vi "Agilent B2900oP AND ip.vi"() -> ()   [LabVIEW 2017]
doc: "This example shows how to configure the instrument's output voltage level, over current protection, and over voltage protection. The actual voltage level and actual current level are returned as well as whether over voltage protection (OVP) or over current protection (OCP) has been tripped."
uses:
  <instrlib>/Agilent B2900 Series/Agilent B2900 Series.lvlib
panel:
  in  "Compliance Voltage (2 V)":dbl=2.0 format="%#_13g"
  in  "Source current (A)":dbl
  in  "Source Range (A)":dbl=2.0
  in  "Enable Output Protection (T: Enable)":bool=TRUE
  in  "Stop":bool
  out "Actual Current Level (A)":dbl format="%_6g"
  out "Actual Voltage Level (V)":dbl format="%_6g"
  in  "VISA resource name":refnum<visa-resource-name>
  # "Compliance Protection"
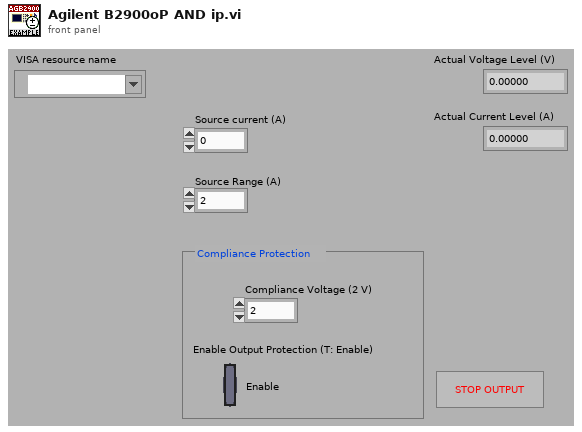
[diagram p1: front panel]
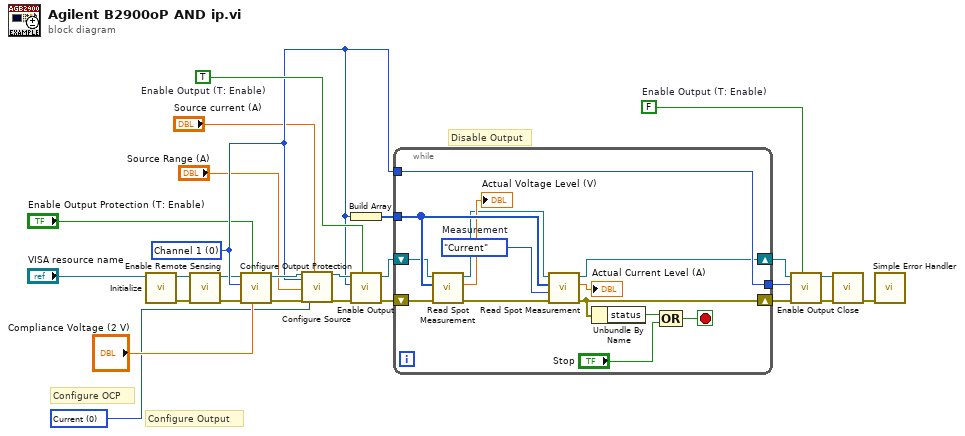
[diagram p0: block diagram]
diagram:
  w10 = 0 items=["Channel 1", "Channel 2"] ("Channel (0: Channel 1)")
  w5 = 0 items=["Current", "Voltage"] ("Source Mode (1: Voltage)")
  w17 = FALSE  # Enable Output (T: Enable)
  w16 = TRUE  # Enable Output (T: Enable)
  # "Disable Output"
  # "Configure Output"
  # "Configure OCP"
  n1 = call <instrlib>:"Initialize.vi"("VISA resource name"="VISA resource name") -> ("error out"=w2:errorcluster, "VISA resource name out"=w4:refnum<visa-resource-name>)  [unwired: 9 in]
  n2 = call <instrlib>:"Enable Remote Sensing.vi"("error in (no error)"=w2, "VISA resource name"=w4) -> ("error out"=w1:errorcluster, "VISA resource name out"=w3:refnum<visa-resource-name>)  [unwired: 8 in]
  n3 = call <instrlib>:"Configure Output Protection.vi"("Compliance Voltage (2 V)"="Compliance Voltage (2 V)", "Enable Output Protection (T: Enable)"="Enable Output Protection (T: Enable)", "error in (no error)"=w1, "Channel (0: Channel 1)"=w10, "VISA resource name"=w3) -> ("error out"=w13:errorcluster, "VISA resource name out"=w14:refnum<visa-resource-name>)  [unwired: 5 in]
  n4 = call <instrlib>:"Configure Source.vi"("VISA resource name"=w14, "Channel (0: Channel 1)"=w10, "Source Range (2)"="Source Range (A)", "error in (no error)"=w13, "Source Mode (1: Voltage)"=w5, "Output Level (0)"="Source current (A)") -> ("VISA resource name out"=w12:refnum<visa-resource-name>, "error out"=w11:errorcluster)  [unwired: 12 in]
  n5 = Build Array(w10) -> (w15:i32[])
  n6 = call <instrlib>:"Enable Output.vi"("Enable Output (T: Enable)"=w16, "error in (no error)"=w11, "Channel (0: Channel 1)"=w10, "VISA resource name"=w12) -> ("error out"=w23:errorcluster, "VISA resource name out"=w24:refnum<visa-resource-name>)  [unwired: 5 in, 1 out]
  n7 = while {
    tunnel: w10 -> [w40]
    tunnel: [w40] -> w22
    shift-right: [w29] -> w21
    shift-left: w23 -> [w28]
    tunnel: w15 -> [w38]
    shift-right: [w39] -> w18
    shift-left: w24 -> [w27]
    stop <- w35 stop-if-true
    w31 = enum16{"Voltage", "Current", "Resistance"}."Current"  # Measurement
    n8 = call <instrlib>:"Read Spot Measurement.vi"("error in (no error)"=w28, "Channel List ({Channel1})"=w38, "VISA resource name"=w27) -> ("error out"=w34:errorcluster, "Measurement Result"=→"Actual Voltage Level (V)":dbl, "VISA resource name out"=w32:refnum<visa-resource-name>)  [unwired: 6 in]
    n9 = call <instrlib>:"Read Spot Measurement.vi"("error in (no error)"=w34, "Measurement Mode (0:Voltage)"=w31, "Channel List ({Channel1})"=w38, "VISA resource name"=w32) -> ("error out"=w29:errorcluster, "Measurement Result"=→"Actual Current Level (A)":dbl, "VISA resource name out"=w39:refnum<visa-resource-name>)  [unwired: 5 in]
    n10 = Unbundle By Name(w29) -> ("status"=w37:bool)
    n11 = Compound Arithmetic op=OR(w37, "Stop") -> (w35:bool)
  }
  n12 = call <instrlib>:"Enable Output.vi"("Enable Output (T: Enable)"=w17, "error in (no error)"=w21, "Channel (0: Channel 1)"=w22, "VISA resource name"=w18) -> ("error out"=w19:errorcluster, "VISA resource name out"=w20:refnum<visa-resource-name>)  [unwired: 5 in, 1 out]
  n13 = call <instrlib>:"Close.vi"("error in (no error)"=w19, "VISA resource name"=w20) -> ("error out"=w25:errorcluster)  [unwired: 9 in]
  n14 = call <vilib>:"Simple Error Handler.vi"("error in (no error)"=w25) -> ()  [unwired: 4 in, 5 out]
